vi "FPGA - Select Bitfile (Local).vi"(8 "error in (no error)":errorcluster, 11 "Node Ptr":u64 format="%.0x") -> (0 "error out":errorcluster)   [LabVIEW 2016, in "Scan Engine Custom Device.lvlib"]
uses:
  Scan Engine Custom Device.lvlib
  Type Defs/FPGA Target.ctl
  <vilib>/NI Veristand/Custom Device Tools/Custom Device Utility Library/Custom Device Utility Library.lvlib
  Type Defs/Host - FPGAScanInterfaceMode.ctl
panel:
  in  "Tag":string
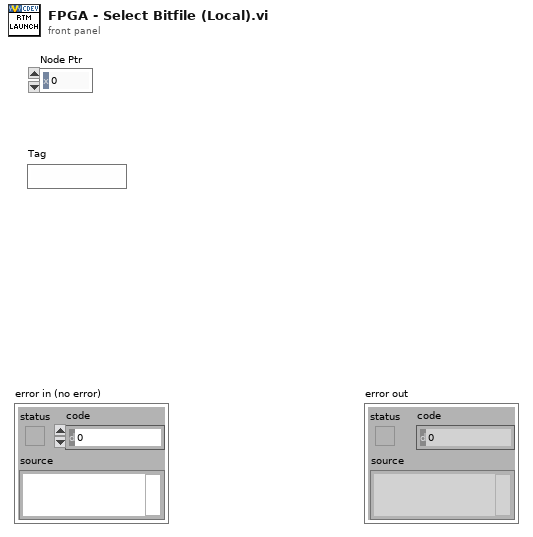
[diagram p1: front panel]
types:
  T1 = typedef "Scan Engine Custom Device.lvlib/Host - FPGAScanInterfaceMode.ctl" = enum16{"Use Current", "FPGA", "Scan Mode"}
  T2 = typedef "Scan Engine Custom Device.lvlib/FPGA Target.ctl" = enum16{"Local", "EtherCAT"}
  T3 = typedef "Custom Device API.lvlib/Custom Device Item Ref.ctl" = u64
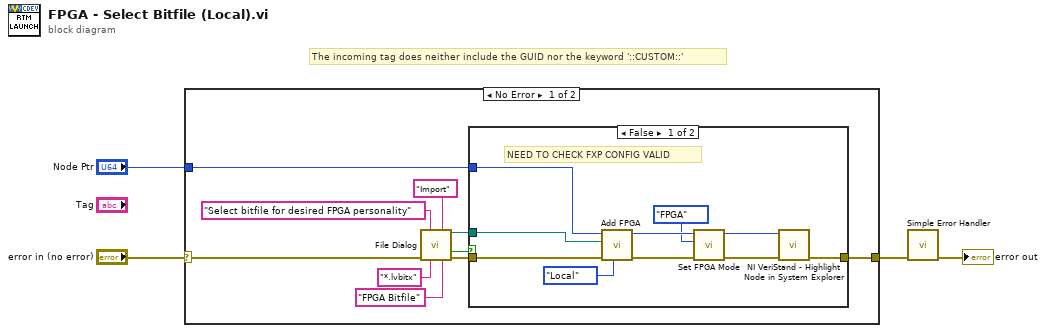
[diagram p0: block diagram]
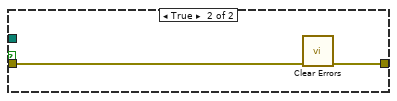
[diagram p2: hidden frame]
diagram:
  # "The incoming tag does neither include the GUID nor the keyword '::CUSTOM::'"
  n1 = case shown="No Error" "error in (no error)" {
    selector: "error in (no error)" -> [w6 w27]
    tunnel: "Node Ptr" -> [w5 _]
    tunnel: [w7 w27] -> w2
    frame No Error {
      n2 = call "File Dialog"("prompt"="Select bitfile for desired FPGA personality", "button label"="Import", "error in"=w6, "pattern (all files)"="*.lvbitx", "pattern label"="FPGA Bitfile") -> ("selected path"=w14:path, "cancelled"=w12:bool, "error out"=w13:errorcluster)  [unwired: 7 in, 1 out]
      n3 = case shown="False" w12 {
        tunnel: w13 -> [w21 w26]
        tunnel: w14 -> [w23 _]
        tunnel: [w20 w25] -> w7
        tunnel: w5 -> [w24 _]
        frame False {
          # "NEED TO CHECK FXP CONFIG VALID"
          n4 = call "Add FPGA.vi"("FPGA Target"=FPGA_Target."Local", "error in (no error)"=w21, "Bitfile Path"=w23, "Item Ref in"=w24) -> ("error out"=w18:errorcluster, "Item Ref out"=w19:T3)  [unwired: 6 in]
          n5 = call "Set FPGA Mode.vi"("error in (no error)"=w18, "FPGAScanInterfaceMode"=Host_-_FPGAScanInterfaceMode."FPGA", "Item Ref in"=w19) -> ("error out"=w15:errorcluster, "Item Ref out"=w16:T3)  [unwired: 7 in]
          n6 = call <vilib>:"NI VeriStand - Highlight Node in System Explorer.vi"("error in (no error)"=w15, "Item Ref in"=w16) -> ("error out"=w20:errorcluster)  [unwired: 8 in, 1 out]
        }
        frame True {
          n7 = call <vilib>:"Clear Errors.vi"("error in (no error)"=w26) -> ("error out"=w25:errorcluster)  [unwired: 1 in, 5 out]
        }
      }
    }
    frame Error {
    }
  }
  n8 = call <vilib>:"Simple Error Handler.vi"("error in (no error)"=w2) -> ("error out"=→"error out":errorcluster)  [unwired: 4 in, 4 out]
